vi "SetWinchPosition.vi"   [LabVIEW 2015]
uses:
  Utilities/MotorPositionGlobals.vi
types:
  T1 = typedef "WPI_MotorControlDeviceRef.ctl" = cluster{"DeviceStatus":errorcluster, "Type":T2, "PWM":cluster{"PWM Channel":T3, "DeadBand":T4}, "CAN":cluster{"Device Number":u8, "Control Mode":T5, "Semaphore":T6, "Max Vout":dbl, "TalonSRX Control Mode":T7}, "Invert":bool}
  T2 = typedef "WPI_MotorControlType.ctl" = enum16{"PWM", "CAN", "CANTalonSRX"}
  T3 = typedef "FPGA_DIOPWMChannel.ctl" = enum8{"PWM 0", "PWM 1", "PWM 2", "PWM 3", "PWM 4", "PWM 5", "PWM 6", "PWM 7", "PWM 8", "PWM 9", "PWM MXP 0", "PWM MXP 1", "PWM MXP 2", "PWM MXP 3", "PWM MXP 4", "PWM MXP 5", "PWM MXP 6", "PWM MXP 7", "PWM MXP 8", "PWM MXP 9", "Invalid"}
  T4 = typedef "WPI_PWMDeadband.ctl" = cluster{"Name":string, "maxPositivePwm":i32, "minPositivePwm":i32, "centerPwm":i32, "maxNegativePwm":i32, "minNegativePwm":i32, "angularRange":u16}
  T5 = typedef "WPI_CANJaguar_ControlMode.ctl" = enum8{"Percent VBus", "Current", "Speed", "Position", "Voltage"}
  T6 = typedef "Semaphore RefNum" = refnum<k1>
  T7 = typedef "WPI_CANTalonSRX_APIControlMode.ctl" = enum8{"Percent VBus", "Speed", "Position", "Slave", "Unchanged / Invalid", "Voltage Compensation", "Current", "Motion Profile"}
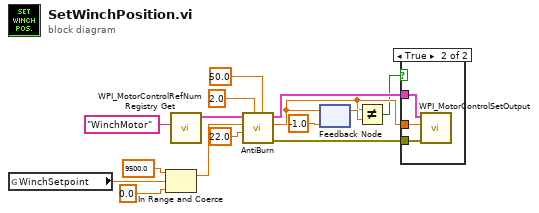
[diagram p0: block diagram]
diagram:
  n1 = global read "MotorPositionGlobals.vi" "WinchSetpoint"() -> (w15:dbl)
  n2 = In Range and Coerce(upper limit=9500.0, x=w15, lower limit=0.0) -> (coerced(x)=w10:dbl)  [unwired: 1 out]
  n3 = call <vilib>:"WPI_MotorControlRefNum Registry Get.vi"("refnum name"="WinchMotor") -> ("MotorControlDevRef"=w1:T1)  [unwired: 9 in, 1 out]
  n4 = call "AntiBurn.vi"("AllowedEncoderError"=50.0, "AllowedTimeDeviation"=2.0, "MaxCurrent"=22.0, "MotorSetpoint"=w10, "CAN Talon SRX Ref"=w1) -> ("error out"=w11:errorcluster, "MotorSetpointOut"=w5:dbl, "MotorControlDevRef"=w12:T1)  [unwired: 3 in, 1 out]
  n5 = feedback-in #1(w5) -> ()
  n6 = feedback #1(-1.0 ("MotorSetpointOut")) -> (w6:dbl)
  n7 = Not Equal?(x=w5, y=w6) -> (x != y?=w3:bool)
  n8 = case shown="True" w3 {
    tunnel: w12 -> [_ w18]
    tunnel: w11 -> [_ w17]
    tunnel: w5 -> [_ w16]
    frame False {
    }
    frame True {
      n9 = call <vilib>:"WPI_MotorControlSetOutput.vi"("error in (no error)"=w17, "Output"=w16, "MotorControlDevRef"=w18) -> ()  [unwired: 6 in, 3 out]
    }
  }
